vi "Add Braces Array.vi"(1 "String in":string[](array[string])) -> (0 "String out":string[](array[string]))   [LabVIEW 2019, in "SMO.Transport.lvclass"]
uses:
  SMO.Transport.lvclass
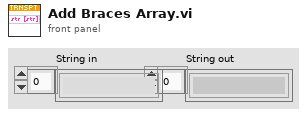
[diagram p1: front panel]
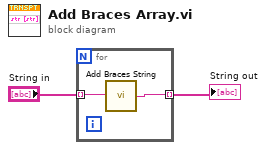
[diagram p0: block diagram]
diagram:
  n1 = for {
    tunnel: "String in" -> [w4] mode=indexing
    tunnel: [w3] -> w1 mode=indexing
    n2 = call "Add Braces String.vi"("String in"=w4) -> ("String out"=w3:string)
  }
  "String out" <- w1
